vi "GetPoint.vi"(7 "Mode":enum16{"Read", "Configure"}(ring), 10 "Settings":T1={"Scan mode"=enum."Points", "NumPoints"=0, "NumReps"=0, "Motion Increment"=0, "NumMotionPoints"=0, "VolumeSettings"={"XStart"=0, "XEnd"=0, "XNum"=1, "YStart"=0, "YEnd"=0, "YNum"=1, "ZStart"=0, "ZEnd"=0, "ZNum"=1}} {"VolumeSettings"."ZNum" min=1 max=10000; "VolumeSettings"."YNum" min=1 max=10000; "VolumeSettings"."XNum" min=1 max=10000}, 11 "Sample Number":u32) -> (0 "RepNum":u32, 1 "Point Num":u32, 2 "Done":bool, 3 "Point":cluster{"X":i32, "Y":i32, "Z":i32})   [LabVIEW 2011]
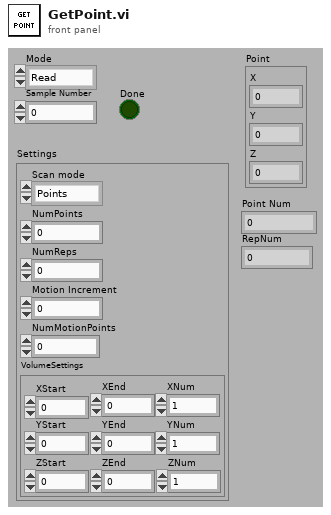
[diagram p1: front panel]
types:
  T1 = cluster{"Scan mode":enum16{"Points", "Volume", "Idle"}, "NumPoints":u32, "NumReps":u32, "Motion Increment":u32, "NumMotionPoints":u32, "VolumeSettings":cluster{"XStart":i32, "XEnd":i32, "XNum":i32, "YStart":i32, "YEnd":i32, "YNum":i32, "ZStart":i32, "ZEnd":i32, "ZNum":i32}}
  T2 = cluster{"XStart":i32, "XEnd":i32, "XNum":i32, "YStart":i32, "YEnd":i32, "YNum":i32, "ZStart":i32, "ZEnd":i32, "ZNum":i32}
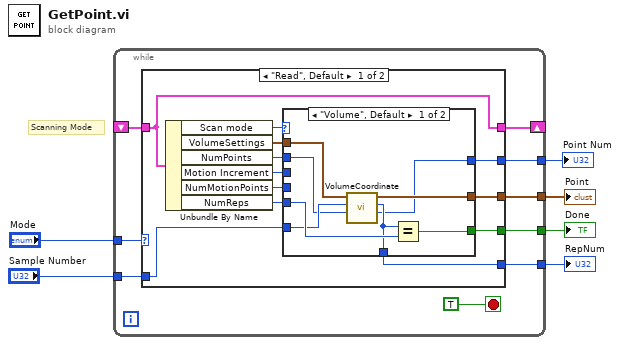
[diagram p0: block diagram]
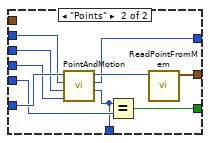
[diagram p2: hidden frame]
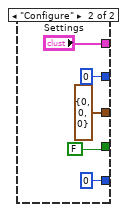
[diagram p3: hidden frame]
diagram:
  # "Scanning Mode"
  n1 = while {
    tunnel: "Mode" -> [w14]
    shift-right: [w13] -> _
    shift-left: _ -> [w12]
    tunnel: "Sample Number" -> [w11]
    tunnel: [w10] -> w4
    tunnel: [w9] -> w3
    tunnel: [w8] -> w2
    tunnel: [w7] -> w1
    stop <- TRUE stop-if-true
    n2 = case shown="\"Read\", Default" w14 {
      tunnel: [w26 "Settings"] -> w13
      tunnel: w12 -> [w26 _]
      tunnel: w11 -> [w27 _]
      tunnel: [w20 cluster{"X":i32, "Y":i32, "Z":i32} {"X"=0, "Y"=0, "Z"=0} ("Point")] -> w10
      tunnel: [w18 FALSE] -> w9
      tunnel: [w17 u32 0 ("Point Num")] -> w8
      tunnel: [w16 u32 0 ("Rep Num")] -> w7
      frame "Read", Default {
        n3 = Unbundle By Name(w26) -> ("Scan mode"=w25:enum16{"Points", "Volume", "Idle"}, "VolumeSettings"=w24:T2, "NumPoints"=w23:u32, "Motion Increment"=w22:u32, "NumMotionPoints"=w21:u32, "NumReps"=w19:u32)
        n4 = case shown="\"Volume\", Default" w25 {
          tunnel: w27 -> [w31 w44]
          tunnel: [w35 w45] -> w20
          tunnel: w24 -> [w34 _]
          tunnel: w23 -> [w28 w43]
          tunnel: w22 -> [_ w42]
          tunnel: w21 -> [_ w41]
          tunnel: w19 -> [w33 w39]
          tunnel: [w32 w38] -> w18
          tunnel: [w29 w37] -> w17
          tunnel: [w30 w36] -> w16
          frame "Volume", Default {
            n5 = call "VolumeCoordinate.vi"("NumPoints"=w28, "SampleNum"=w31, "Scan Settings"=w34) -> ("PointNum"=w29:u32, "RepNum"=w30:u32, "Point"=w35:cluster{"X":i32, "Y":i32, "Z":i32})  [unwired: 6 in]
            n6 = Equal?(x=w30, y=w33) -> (x = y?=w32:bool)
          }
          frame "Points" {
            n7 = call "PointAndMotion.vi"("Motion Points"=w41, "Motion Increment"=w42, "Num Points"=w43, "Sample Num"=w44) -> ("Rep Num"=w36:u32, "Point Num"=w37:u32, "Point Location"=w40:u32)  [unwired: 4 in, 1 out]
            n8 = Equal?(x=w36, y=w39) -> (x = y?=w38:bool)
            n9 = call "ReadPointFromMem.vi"("PointNum"=w40) -> ("Point"=w45:cluster{"X":i32, "Y":i32, "Z":i32})  [unwired: 10 in]
          }
        }
      }
      frame "Configure" {
      }
    }
  }
  "Point" <- w4
  "Done" <- w3
  "Point Num" <- w2
  "RepNum" <- w1
